vi "Update Status.vi"(9 "ID":i32, 10 "MyPosition":cluster{"X":i32, "Y":i32}, 11 "Mother in":refnum<class "Formics.lvclass">) -> (3 "Mother out":refnum<class "Formics.lvclass">)   [LabVIEW 2014, in "Formics.lvclass"]
uses:
  Formics.lvclass
  Formics.lvclass/Formics.ctl
  SquareStatus.ctl
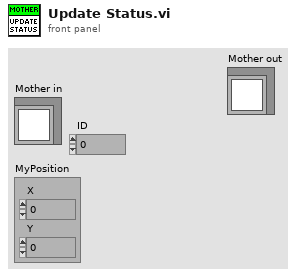
[diagram p1: front panel]
types:
  T1 = typedef "Formics.lvclass/SquareStatus DVR.ctl" = refnum<data-value>
  T2 = typedef "Formics.lvclass/SquareStatus.ctl" = cluster{"ID":i32, "Heartbeat":bool}
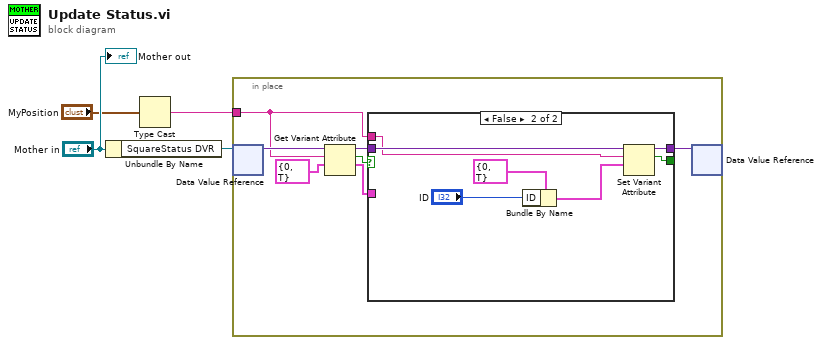
[diagram p0: block diagram]
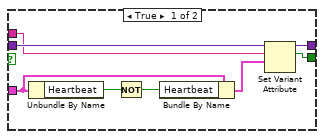
[diagram p2: hidden frame]
diagram:
  n1 = Unbundle By Name("Mother in") -> ("SquareStatus DVR"=w1:T1)
  n2 = Type Cast(x="MyPosition") -> (*(type *) &x=w3:string)  [unwired: 1 in]
  n3 = in-place {
    in-place-border: w3 -> [w5]
    n4 = in-place-dvr #1(w1) -> (w10:variant)  [unwired: 1 out]
    n5 = Get Variant Attribute(Variant=w10, name=w5, default value (empty Variant)=T2 {"ID"=0, "Heartbeat"=TRUE} ("Shared Info")) -> (duplicate Variant=w9:variant, found=w7:bool, value=w6:T2)  [unwired: 1 in, 1 out]
    n6 = case shown="False" w7 {
      tunnel: [w19 w26] -> w8
      tunnel: [w18 w25] -> _
      tunnel: w9 -> [w15 w24]
      tunnel: w6 -> [w13 _]
      tunnel: w5 -> [w12 w23]
      frame True {
        n7 = Unbundle By Name(w13) -> ("Heartbeat"=w17:bool)
        n8 = Not(x=w17) -> (.not. x?=w16:bool)
        n9 = Bundle By Name(cluster=w13, "Heartbeat"=w16) -> (w14:T2)
        n10 = Set Variant Attribute(Variant=w15, name=w12, value=w14) -> (Variant out=w19:variant, replaced=w18:bool)  [unwired: 1 in, 1 out]
      }
      frame False {
        n11 = Bundle By Name(cluster=T2 {"ID"=0, "Heartbeat"=TRUE} ("Shared Info"), "ID"="ID") -> (w21:T2)
        n12 = Set Variant Attribute(Variant=w24, name=w23, value=w21) -> (Variant out=w26:variant, replaced=w25:bool)  [unwired: 1 in, 1 out]
      }
    }
    n13 = in-place-dvr #1(w8) -> ()  [unwired: 2 out]
  }
  "Mother out" <- "Mother in"
